vi "Test.vi"() -> ()   [LabVIEW 2014]
uses:
  TypeDefs/mObject.ctl
  TypeDefs/BG Image.ctl
  TypeDefs/Mimic Data.ctl
  <vilib>/Utility/miscctls.llb/LVPointTypeDef.ctl
  MATH/MathLoop/TypeDefs/ParsedExpression.ctl
  MATH/MathLoop/TypeDefs/typeMed.ctl
  MATH/MathLoop/TypeDefs/Conf. Gral.ctl
  Mimico Display.lvlib
  MATH/MathLoop/MathLoop.lvlib
panel:
  out "Mimic Picture 2":picture
  out "Array":sgl[](array[numeric])
  out "picture out":picture
  in  "stop 3":bool
  in  "DEL":bool
  in  "ADD":bool
  in  "BG Image":T1={"Path"=path "\\\\VBOXSVR\\e_drive/Repositorio MAGNIS/INF002/v0/Modules/SEQ/Mimico Display/PTGM0003-00093281952.bmp", "point"={"x"=0, "y"=0}}
  in  "mObject Data":T2
  in  "Mediciones  Disponibles":i32(listbox)
  in  "stop":bool
  out "Mimic Picture":picture
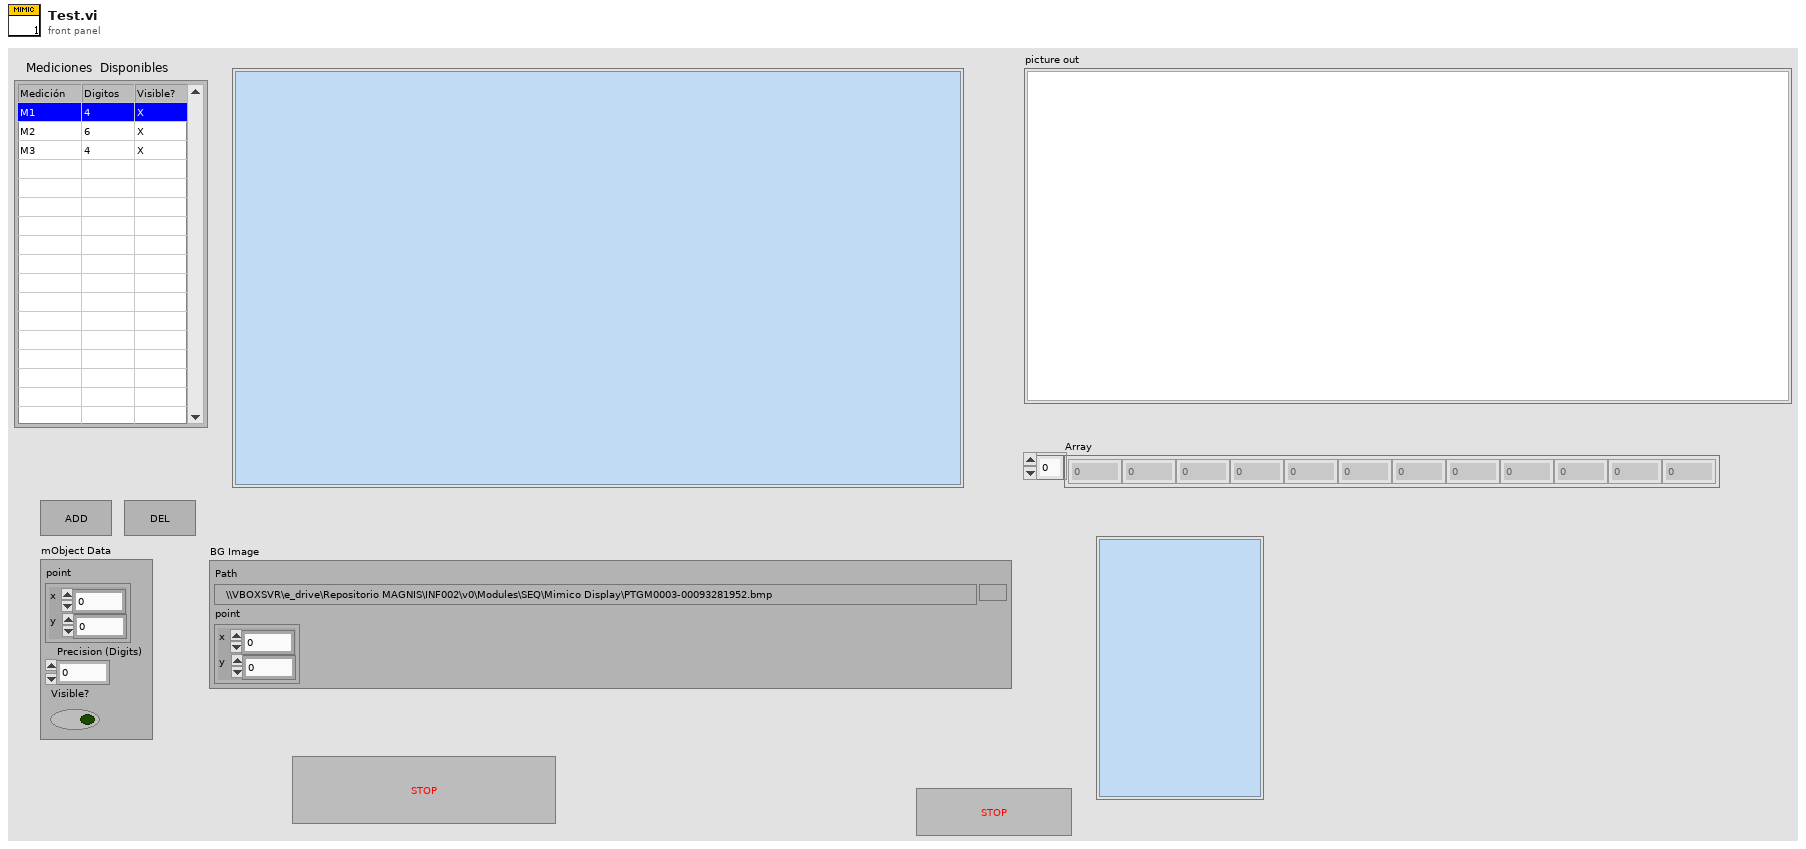
[diagram p1: front panel]
types:
  T1 = typedef "BG Image.ctl" = cluster{"Path":path, "point":cluster{"x":i16, "y":i16}}
  T2 = typedef "mObject.ctl" = cluster{"point":cluster{"x":i16, "y":i16}, "Precision (Digits)":i32, "Visible?":bool}
  T3 = typedef "MathLoop.lvlib/ParsedExpression.ctl" = cluster{"RPN ":string[], "Constantes":sgl[], "Variables":string[], "Formula":string, "Tipo de Med":T4, "Med?":bool, "Descripción":string, "Nominal":sgl, "Tol Sup":sgl, "Pre TS":sgl, "Pre TI":sgl, "Tol Inf":sgl}
  T4 = typedef "MathLoop.lvlib/typeMed.ctl" = string
  T5 = typedef "MathLoop.lvlib/Conf. Gral.ctl" = cluster{"Engranometro":cluster{"Cant. Dientes x pieza":i32, "Nro. Dientes (Frp)":i32, "Armonicas":i32}}
  T6 = cluster{"Variable Data Out":cluster{"Kcte":sgl[], "Dcte":sgl[], "Aux":sgl[][], "Transductores":sgl[][]}, "Array":sgl[], T3[], "Array Med":sgl[][], "Conf. General":T5}
  T7 = typedef "LVPointTypeDef.ctl" = cluster{"Horizontal":i16, "Vertical":i16}
  T8 = typedef "Mimico Display.lvlib/Mimic Data.ctl" = cluster{"BG Image":T1, "Mimic mObjects":T2[], "Mimic Picture":picture}
  T9 = typedef "eventvkey.ctl" = enum16{"ASCII", "Enter", "Return", "Shift", "Ctrl", "Alt", "Cmd", "Opt", "Caps", "NumLock", "Clear", "Break", "Up", "Down", "Left", "Right", "Insert", "Delete", "Home", "End", "PageUp", "PageDown", "Escape", "Help", "Pause", "ScrollLock", "F1", "F2", "F3", "F4", "F5", "F6", "F7", "F8", "F9", "F10", "F11", "F12", "F13", "F14", "F15", "F16", "F17", "F18", "F19", "F20", "F21", "F22", "F23", "F24", "Play", "VolumeUp", "VolumeDown", "Mute", "Two Byte Char"}
  T10 = typedef "LVMouseTypeDef.ctl" = cluster{"Mouse Position":cluster{"X":i32, "Y":i32}, "Mouse Modifiers":cluster{"Button Down":bool, "Shift Mod":bool, "Menu Mod":bool, "Option Mod":bool}}
  T11 = cluster{"Descripción":string, "Nominal":sgl, "Tol Sup":sgl, "Pre TS":sgl, "Pre TI":sgl, "Tol Inf":sgl}
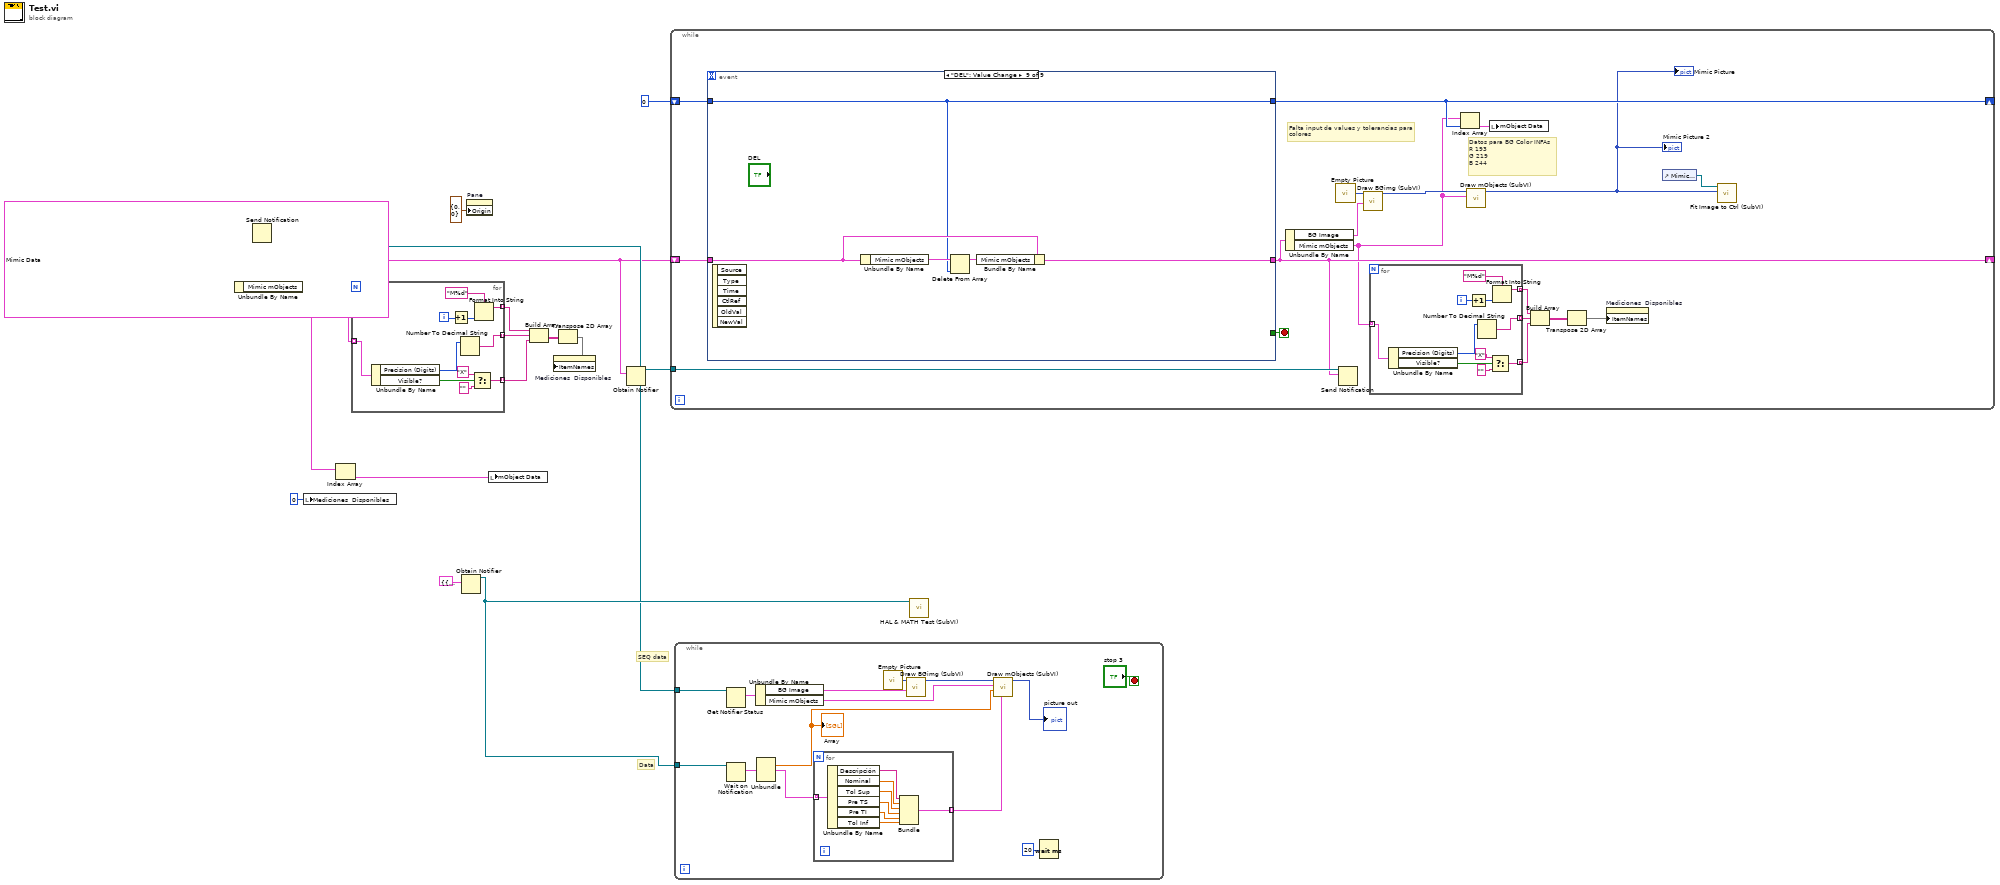
[diagram p0: block diagram]
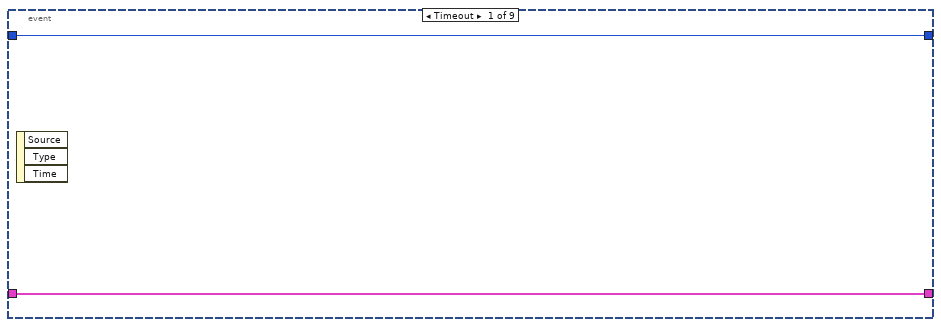
[diagram p2: hidden frame]
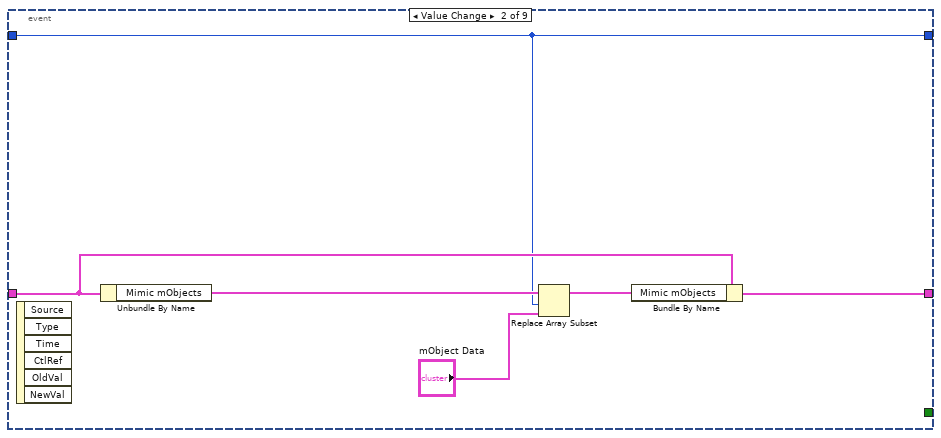
[diagram p3: hidden frame]
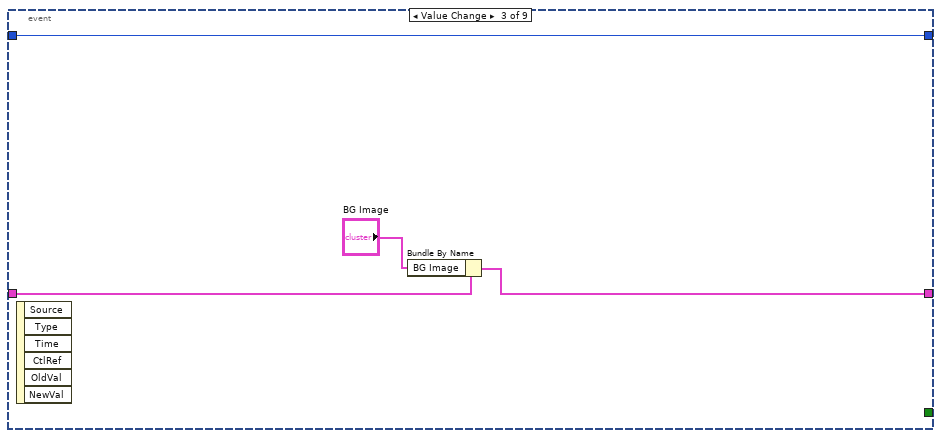
[diagram p4: hidden frame]
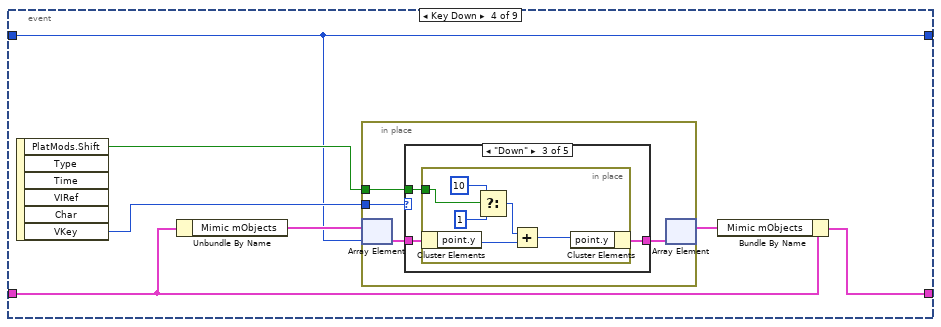
[diagram p5: hidden frame]
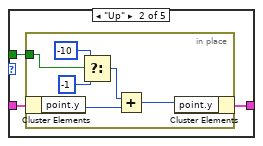
[diagram p7: hidden frame]
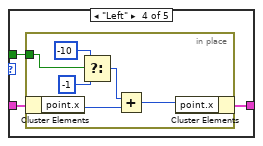
[diagram p8: hidden frame]
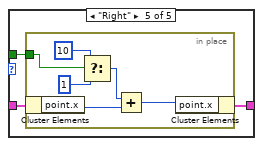
[diagram p9: hidden frame]
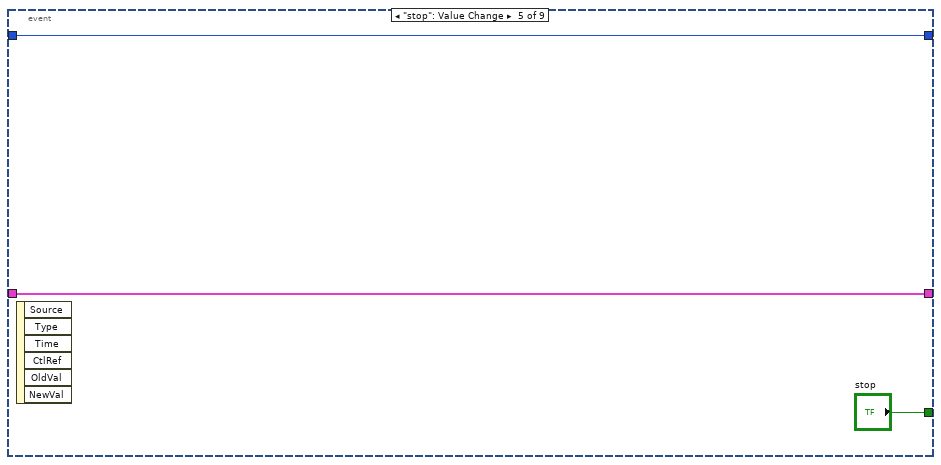
[diagram p10: hidden frame]
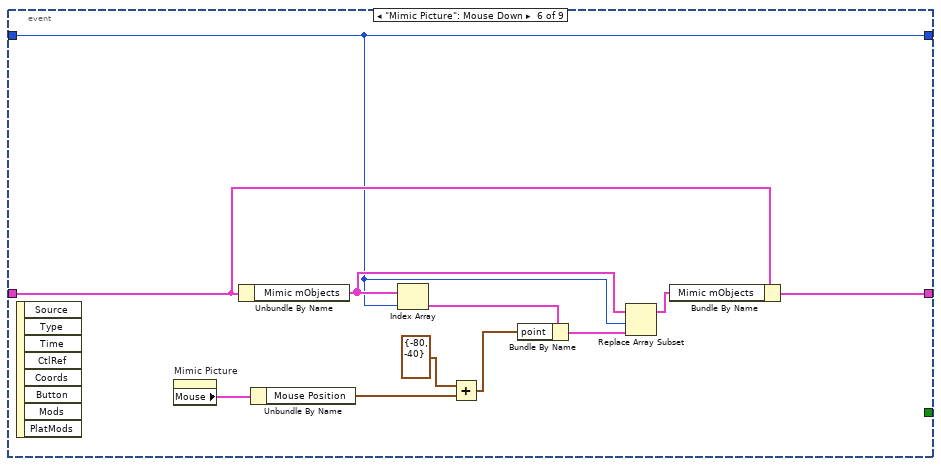
[diagram p11: hidden frame]
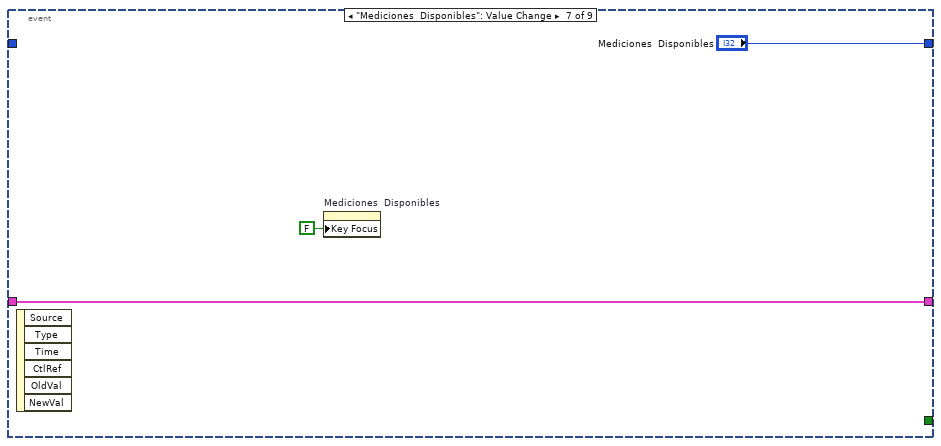
[diagram p12: hidden frame]
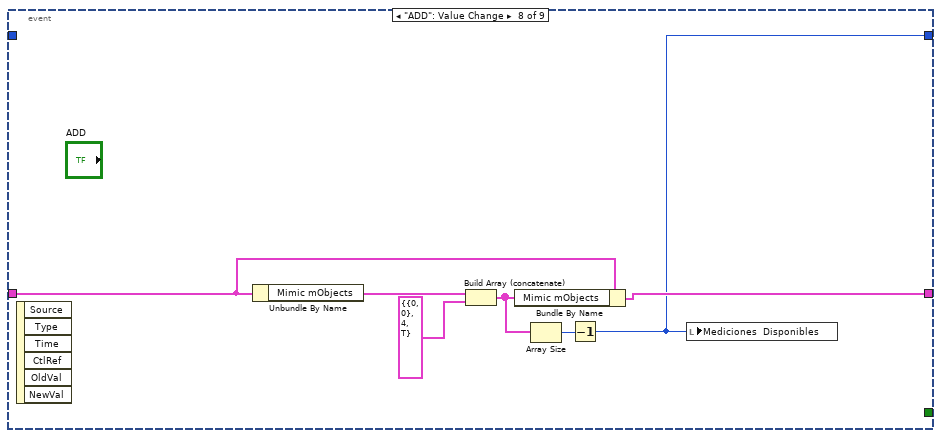
[diagram p13: hidden frame]
diagram:
  w7 = T8 {"BG Image"={"Path"=path "\\\\VBOXSVR\\e_drive/Repositorio MAGNIS/INF002/v0/Modules/SEQ/Mimico Display/PTGM0003-00093281952.bmp", "point"={"x"=0, "y"=0}}, "Mimic mObjects"=[{"point"={"x"=100, "y"=100}, "Precision (Digits)"=4, "Visible?"=TRUE}, {"point"={"x"=100, "y"=300}, "Precision (Digits)"=6, "Visible?"=TRUE}, {"point"={"x"=300, "y"=100}, "Precision (Digits)"=4, "Visible?"=TRUE}], "Mimic Picture"=bytes[0]} ("Mimic Data")
  # "Data"
  # "SEQ data"
  n1 = Unbundle By Name(w7) -> ("Mimic mObjects"=w6:T2[])
  n2 = local write "Mediciones  Disponibles"(0 ("Mediciones  Disponibles")) -> ()
  n3 = Index Array(array=w6) -> (element=w13:T2)  [unwired: 1 in]
  n4 = for {
    tunnel: [w22] -> w5 mode=indexing
    tunnel: w6 -> [w21] mode=indexing
    tunnel: [w20] -> w4 mode=indexing
    tunnel: [w15] -> w3 mode=indexing
    i -> [w24]
    n5 = Unbundle By Name(w21) -> ("Precision (Digits)"=w19:i32, "Visible?"=w18:bool)
    n6 = Increment(x=w24) -> (x+1=w25:i32)
    n7 = Number To Decimal String(number=w19) -> (decimal integer string=w20:string)  [unwired: 1 in]
    n8 = Select(t="X" ("format string"), s=w18, f="" ("format string")) -> (s? t:f=w15:string)
    n9 = Format Into String(format string="M%d", w25) -> (resulting string=w22:string)  [unwired: 2 in, 1 out]
  }
  n10 = Obtain Notifier(notification data type=T6 {"Variable Data Out"={"Kcte"=[], "Dcte"=[], "Aux"=[], "Transductores"=[]}, "Array"=[], [], "Array Med"=[], "Conf. General"={"Engranometro"={"Cant. Dientes x pieza"=0, "Nro. Dientes (Frp)"=0, "Armonicas"=0}}} ("output cluster")) -> (notifier out=w9:refnum<notifier>)  [unwired: 3 in, 2 out]
  n11 = property on="Pane" class="Pane"("Origin"=T7 {"Horizontal"=0, "Vertical"=0}) -> ()  [unwired: 2 in, 2 out]
  n12 = local write "mObject Data"(w13) -> ()
  n13 = Build Array(w5, w4, w3) -> (w2:string[][])
  n14 = Transpose 2D Array(2D array=w2) -> (transposed array=w1:string[][])
  n15 = property on="Mediciones  Disponibles" class="MCListbox (strict)"("ItemNames"=w1) -> ()  [unwired: 2 in, 2 out]
  n16 = Obtain Notifier(notification data type=w7) -> (notifier out=w8:refnum<notifier>)  [unwired: 3 in, 2 out]
  n17 = Send Notification(notification=w7, notifier=w8) -> ()  [unwired: 1 in, 2 out]
  n18 = while {
    shift-right: [w34] -> _
    shift-left: w7 -> [w43]
    shift-right: [w36] -> _
    shift-left: 0 ("Mediciones  Disponibles") -> [w37]
    tunnel: w8 -> [w35]
    stop <- w39 stop-if-true
    # "Datos para BG Color INFAs\nR 193\nG 219\nB 244"
    # "Falta input de values y tolerancias para\ncolores"
    n19 = event shown="[8] \"DEL\": Value Change" {
      selector: _ -> [_ _ _ _ _ _ _ _ _]
      dyn-events: _ -> [_ _ _ _ _ _ _ _ _]
      timeout: _ -> [_ _ _ _ _ _ _ _ _]
      tunnel: w43 -> [w56 w62 w65 w73 w117 w127 w131 w136 w141]
      tunnel: [w56 w58 w64 w69 w117 w123 w131 w135 w140] -> w34
      tunnel: [_ _ _ _ "stop" _ _ _ _] -> w39
      tunnel: w37 -> [w55 w57 w63 w67 w115 w121 _ _ w139]
      tunnel: [w55 w57 w63 w67 w115 w121 "Mediciones  Disponibles" w132 w139] -> w36
      event Timeout {
        n20 = event-data() -> ()  [unwired: 1 in, 3 out]
      }
      event Value Change {
        n21 = event-data() -> ()  [unwired: 1 in, 6 out]
        n22 = Unbundle By Name(w62) -> ("Mimic mObjects"=w61:T2[])
        n23 = Replace Array Subset(array=w61, new element="mObject Data", index=w57) -> (w59:T2[])
        n24 = Bundle By Name(cluster=w62, "Mimic mObjects"=w59) -> (w58:T8)
      }
      event Value Change {
        n25 = event-data() -> ()  [unwired: 1 in, 6 out]
        n26 = Bundle By Name(cluster=w65, "BG Image"="BG Image") -> (w64:T8)
      }
      event Key Down {
        n27 = event-data() -> ("PlatMods.Shift"=w68:bool, "VKey"=w72:T9)  [unwired: 1 in, 4 out]
        n28 = Unbundle By Name(w73) -> ("Mimic mObjects"=w71:T2[])
        n29 = in-place {
          in-place-border: w72 -> [w77]
          in-place-border: w68 -> [w74]
          n30 = in-place-array #1(w71, w67) -> (w76:T2)
          n31 = case shown="\"Down\"" w77 {
            tunnel: w76 -> [w78 w81 w90 w99 w108]
            tunnel: [w78 w80 w89 w98 w107] -> w75
            tunnel: w74 -> [_ w79 w88 w97 w106]
            frame Default {
            }
            frame "Up" {
              n32 = in-place {
                in-place-border: w79 -> [w84]
                n33 = in-place-cluster #2(w81) -> ("point.y"=w87:i16)
                n34 = Select(t=-10, s=w84, f=-1) -> (s? t:f=w85:i32)
                n35 = Add(x=w85, y=w87) -> (x+y=w86:i32)
                n36 = in-place-cluster #2("point.y"=w86) -> (w80:T2)
              }
            }
            frame "Down" {
              n37 = in-place {
                in-place-border: w88 -> [w93]
                n38 = in-place-cluster #3(w90) -> ("point.y"=w96:i16)
                n39 = Select(t=10, s=w93, f=1) -> (s? t:f=w94:i32)
                n40 = Add(x=w94, y=w96) -> (x+y=w95:i32)
                n41 = in-place-cluster #3("point.y"=w95) -> (w89:T2)
              }
            }
            frame "Left" {
              n42 = in-place {
                in-place-border: w97 -> [w102]
                n43 = in-place-cluster #4(w99) -> ("point.x"=w105:i16)
                n44 = Select(t=-10, s=w102, f=-1) -> (s? t:f=w103:i32)
                n45 = Add(x=w103, y=w105) -> (x+y=w104:i32)
                n46 = in-place-cluster #4("point.x"=w104) -> (w98:T2)
              }
            }
            frame "Right" {
              n47 = in-place {
                in-place-border: w106 -> [w111]
                n48 = in-place-cluster #5(w108) -> ("point.x"=w114:i16)
                n49 = Select(t=10, s=w111, f=1) -> (s? t:f=w112:i32)
                n50 = Add(x=w112, y=w114) -> (x+y=w113:i32)
                n51 = in-place-cluster #5("point.x"=w113) -> (w107:T2)
              }
            }
          }
          n52 = in-place-array #1(w75) -> (w70:T2[])  [unwired: 1 out]
        }
        n53 = Bundle By Name(cluster=w73, "Mimic mObjects"=w70) -> (w69:T8)
      }
      event "stop": Value Change {
        n54 = event-data() -> ()  [unwired: 1 in, 6 out]
      }
      event "Mimic Picture": Mouse Down {
        n55 = event-data() -> ()  [unwired: 1 in, 8 out]
        n56 = property on="Mimic Picture" class="Pict"() -> ("Mouse"=w128:T10)  [unwired: 2 in, 2 out]
        n57 = Unbundle By Name(w127) -> ("Mimic mObjects"=w125:T2[])
        n58 = Unbundle By Name(w128) -> ("Mouse Position"=w120:cluster{"X":i32, "Y":i32})
        n59 = Index Array(array=w125, index=w121) -> (element=w126:T2)
        n60 = Add(x=cluster{"X":i32, "Y":i32} {"X"=-80, "Y"=-40}, y=w120) -> (x+y=w119:cluster{"X":i32, "Y":i32})
        n61 = Bundle By Name(cluster=w126, "point"=w119) -> (w122:T2)
        n62 = Replace Array Subset(array=w125, new element=w122, index=w121) -> (w124:T2[])
        n63 = Bundle By Name(cluster=w127, "Mimic mObjects"=w124) -> (w123:T8)
      }
      event "Mediciones  Disponibles": Value Change {
        n64 = event-data() -> ()  [unwired: 1 in, 6 out]
        n65 = property on="Mediciones  Disponibles" class="MCListbox (strict)"("Key Focus"=FALSE) -> ()  [unwired: 2 in, 2 out]
      }
      event "ADD": Value Change {
        n66 = event-data() -> ()  [unwired: 1 in, 6 out]
        n67 = Unbundle By Name(w136) -> ("Mimic mObjects"=w138:T2[])
        n68 = Build Array (concatenate)(w138, T2 {"point"={"x"=0, "y"=0}, "Precision (Digits)"=4, "Visible?"=TRUE} ("mObject Data")) -> (w134:T2[])
        n69 = Bundle By Name(cluster=w136, "Mimic mObjects"=w134) -> (w135:T8)
        n70 = Array Size(array=w134) -> (size(s)=w133:i32)
        n71 = Decrement(x=w133) -> (x-1=w132:i32)
        n72 = local write "Mediciones  Disponibles"(w132) -> ()
      }
      event "DEL": Value Change {
        n73 = event-data() -> ()  [unwired: 1 in, 6 out]
        n74 = Unbundle By Name(w141) -> ("Mimic mObjects"=w143:T2[])
        n75 = Delete From Array(array=w143, index=w139) -> (array with subset deleted=w142:T2[])  [unwired: 1 in, 1 out]
        n76 = Bundle By Name(cluster=w141, "Mimic mObjects"=w142) -> (w140:T8)
      }
    }
    n77 = Unbundle By Name(w34) -> ("BG Image"=w40:T1, "Mimic mObjects"=w31:T2[])
    n78 = call "Empty Picture"() -> ("empty picture"=w42:picture)
    n79 = Send Notification(notification=w34, notifier=w35) -> ()  [unwired: 1 in, 2 out]
    n80 = call "Draw BGimg (SubVI).vi"("BG Image"=w40, "picture in"=w42) -> ("picture out"=w41:picture)  [unwired: 9 in]
    n81 = for {
      tunnel: [w51] -> w33 mode=indexing
      tunnel: w31 -> [w50] mode=indexing
      tunnel: [w49] -> w30 mode=indexing
      tunnel: [w44] -> w29 mode=indexing
      i -> [w53]
      n82 = Unbundle By Name(w50) -> ("Precision (Digits)"=w48:i32, "Visible?"=w47:bool)
      n83 = Increment(x=w53) -> (x+1=w54:i32)
      n84 = Number To Decimal String(number=w48) -> (decimal integer string=w49:string)  [unwired: 1 in]
      n85 = Select(t="X" ("format string"), s=w47, f="" ("format string")) -> (s? t:f=w44:string)
      n86 = Format Into String(format string="M%d", w54) -> (resulting string=w51:string)  [unwired: 2 in, 1 out]
    }
    n87 = Index Array(array=w31, index=w36) -> (element=w38:T2)
    n88 = call "Draw mObjects (SubVI).vi"("Mimic mObjects"=w31, "picture in"=w41) -> ("picture out"=w26:picture)  [unwired: 9 in]
    "Mimic Picture" <- w26
    "Mimic Picture 2" <- w26
    n89 = local write "mObject Data"(w38) -> ()
    n90 = Build Array(w33, w30, w29) -> (w28:string[][])
    n91 = Transpose 2D Array(2D array=w28) -> (transposed array=w32:string[][])
    n92 = property on="Mediciones  Disponibles" class="MCListbox (strict)"("ItemNames"=w32) -> ()  [unwired: 2 in, 2 out]
    n93 = control-ref of="Mimic Picture 2"() -> (w27:refnum<vi>)
    n94 = call "Fit Image to Ctrl (SubVI).vi"("picture in"=w26, "Picture ref in"=w27) -> ()  [unwired: 10 in]
  }
  n95 = while {
    tunnel: w8 -> [w153]
    tunnel: w9 -> [w154]
    stop <- "stop 3" stop-if-true
    n96 = Get Notifier Status(notifier=w153) -> (current notification=w151:T8)  [unwired: 1 in, 4 out]
    n97 = Wait on Notification(notifier=w154) -> (notification=w152:T6)  [unwired: 3 in, 3 out]
    n98 = Unbundle By Name(w151) -> ("BG Image"=w150:T1, "Mimic mObjects"=w148:T2[])
    n99 = Unbundle(w152) -> ("Array"=w145:sgl[], w149:T3[])  [unwired: 3 out]
    "Array" <- w145
    n100 = for {
      tunnel: w149 -> [w165] mode=indexing
      tunnel: [w160] -> w146 mode=indexing
      n101 = Unbundle By Name(w165) -> ("Descripción"=w159:string, "Nominal"=w158:sgl, "Tol Sup"=w164:sgl, "Pre TS"=w163:sgl, "Pre TI"=w162:sgl, "Tol Inf"=w161:sgl)
      n102 = Bundle("Descripción"=w159, "Nominal"=w158, "Tol Sup"=w164, "Pre TS"=w163, "Pre TI"=w162, "Tol Inf"=w161) -> (w160:T11)  [unwired: 1 in]
    }
    n103 = call "Empty Picture"() -> ("empty picture"=w156:picture)
    n104 = call "Draw BGimg (SubVI).vi"("BG Image"=w150, "picture in"=w156) -> ("picture out"=w155:picture)  [unwired: 9 in]
    n105 = call "Draw mObjects (SubVI).vi"("Array"=w146, "Math Values (Temporal)"=w145, "Mimic mObjects"=w148, "picture in"=w155) -> ("picture out"=→"picture out":picture)  [unwired: 7 in]
    n106 = Wait (ms)(milliseconds to wait=u32 20) -> ()  [unwired: 1 out]
  }
  n107 = call "HAL & MATH Test (SubVI).vi"("Notifier in"=w9) -> ()  [unwired: 11 in]
